vi "VISA name translate.vi"(0 "Primary Address":u16, 1 "Secondary Address":u16, 3 "board":u16, 4 "Interface":enum16{"GPIB", "Serial"}(ring)) -> (5 "VISA resource name output":refnum<visa-resource-name>)   [LabVIEW 2024]
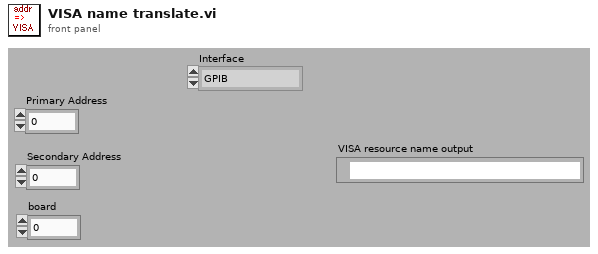
[diagram p1: front panel]
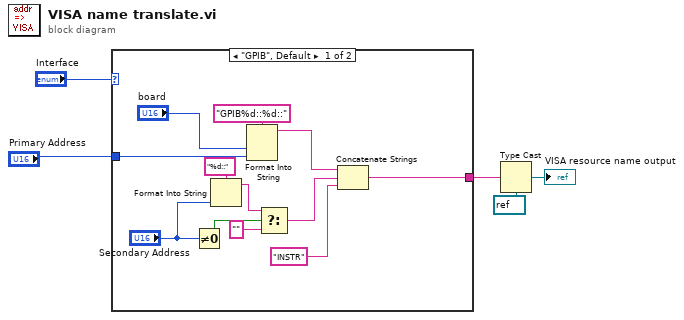
[diagram p0: block diagram]
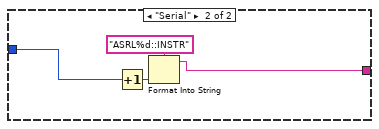
[diagram p2: hidden frame]
diagram:
  n1 = case shown="\"GPIB\", Default" "Interface" {
    tunnel: "Primary Address" -> [w15 w18]
    tunnel: [w9 w19] -> w1
    frame "GPIB", Default {
      n2 = Not Equal To 0?(x="Secondary Address") -> (x != 0?=w14:bool)
      n3 = Format Into String(format string="%d::" ("Format String"), "Secondary Address") -> (resulting string=w6:string)  [unwired: 2 in, 1 out]
      n4 = Format Into String(format string="GPIB%d::%d::" ("Format String"), "board", w15) -> (resulting string=w12:string)  [unwired: 2 in, 1 out]
      n5 = Select(t=w6, s=w14, f="") -> (s? t:f=w11:string)
      n6 = Concatenate Strings(w12, w11, "INSTR" ("Format String")) -> (w9:string)
    }
    frame "Serial" {
      n7 = Increment(x=w18) -> (x+1=w20:u16)
      n8 = Format Into String(format string="ASRL%d::INSTR" ("Format String"), w20) -> (resulting string=w19:string)  [unwired: 2 in, 1 out]
    }
  }
  n9 = Type Cast(type=refnum<visa-resource-name> refnum ("VISA resource name"), x=w1) -> (*(type *) &x=→"VISA resource name output":refnum<visa-resource-name>)
